vi "sig.end_protected_lua.vi"(5 "LuaVIEW reference":T1) -> (15 "error out":errorcluster)   [LabVIEW 2012]
doc: "End a protected section of code. No signals are handled while executing a protected section. This prevents the protected section from being interrupted by anything other than an error. Each call to \"end_protected\" must be preceeded by a matching call to \"begin_protected\". Signals that arrive while executing the protected sections are not discarded, their handling is merely postponed. It is possible to nest protected sections or call functions with protected sections from within a protected section. Signal handling is reenabled only after the outermost \"end_protected\" call.\nErrors:\nMore calls to \"end_protected\" than \"begin_protected\" were made.\nFunction must be called from a task context but was not."
uses:
  typedefs/t_LuaVIEW Reference.ctl
  typedefs/t_LuaVIEW Task State Methods.ctl
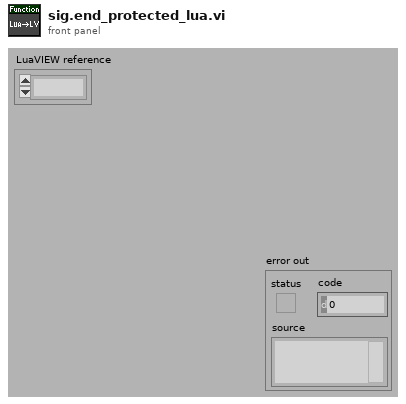
[diagram p1: front panel]
types:
  T1 = typedef "t_LuaVIEW Reference.ctl" = refnum<k1>
  T2 = typedef "t_LuaVIEW Task State Methods.ctl" = enum16{"cleanup", "set initial", "set mode", "set active mode", "set error", "get task info", "get script info", "set signal", "clear signal", "test handled", "test delegated", "test signal", "handle signal", "delegate signal", "allow signal", "disallow signal", "disallow all", "signals?", "delegated signals?", "protection++", "protection--", "protection=0", "message", "next message", "pop message", "message available?", "force stop", "set swap preps", "apply swap preps"}
  T3 = typedef "t_LuaVIEW Task State Pane.ctl" = refnum<vi>
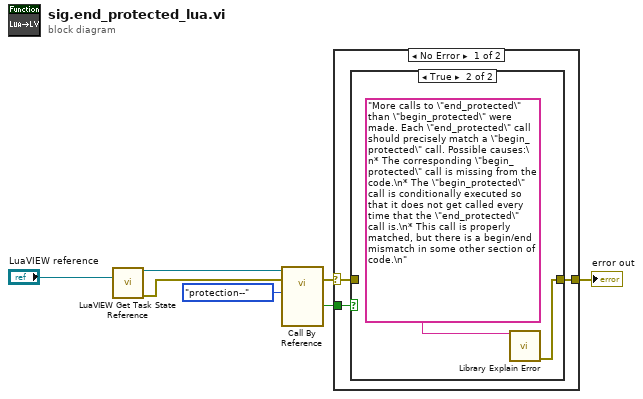
[diagram p0: block diagram]
diagram:
  n1 = call "LuaVIEW Get Task State Reference.vi"("LuaVIEW reference in"="LuaVIEW reference") -> ("task state reference"=w7:T3, "error out"=w4:errorcluster)  [unwired: 12 in, 1 out]
  n2 = call-by-ref "?"(reference=w7, error in=w4, "method"=t_LuaVIEW_Task_State_Methods."protection--") -> (error out=w3:errorcluster, "set/available/pending"=w1:bool)  [unwired: 10 in, 5 out]
  n3 = case shown="No Error" w3 {
    selector: w3 -> [w8 w14]
    tunnel: [w10 w14] -> w2
    tunnel: w1 -> [w9 _]
    frame No Error {
      n4 = case shown="True" w9 {
        tunnel: [w11 w13] -> w10
        tunnel: w8 -> [w11 _]
        frame False {
        }
        frame True {
          n5 = call "Library Explain Error.vi"("explanation prefix (none)"="More calls to \"end_protected\" than \"begin_protected\" were made. Each \"end_protected\" call should precisely match a \"begin_protected\" call. Possible causes:\n* The corresponding \"begin_protected\" call is missing from the code.\n* The \"begin_protected\" call is conditionally executed so that it does not get called every time that the \"end_protected\" call is.\n* This call is properly matched, but there is a begin/end mismatch in some other section of code.\n" ("explanation")) -> ("explained error"=w13:errorcluster)  [unwired: 14 in]
        }
      }
    }
    frame Error {
    }
  }
  "error out" <- w2
